vi "Autonomous Independent.vi"() -> ()   [LabVIEW 2015]
doc: "This VI is called when autonomous begins, and will automatically be terminated when autonomous ends. You can carry out timed or sensor driven robot movement independently without needing to return to the caller."
uses:
  <vilib>/Rock Robotics/WPI/Relay/WPI_RelayValue.ctl
  <vilib>/Rock Robotics/Network Tables/NT Read String.vi
  Robot Global Data.vi
  navX Library v2/navX Library v2.lvlib
panel:
  in  "Routine 2 - Shoot Encoder 2":dbl=1.78
  in  "Routine 2 - Shoot Encoder":dbl=1.78
  in  "Routine 1 - Target Angle":dbl=58.0
  in  "Routine 1 - Shoot Distance":dbl=16.0
  in  "Low Bar Height":dbl=1.2
  in  "Routine 1 - Shoot Encoder":dbl=1.63
  # "Actual distance for routine 1 is 17.5 ft"
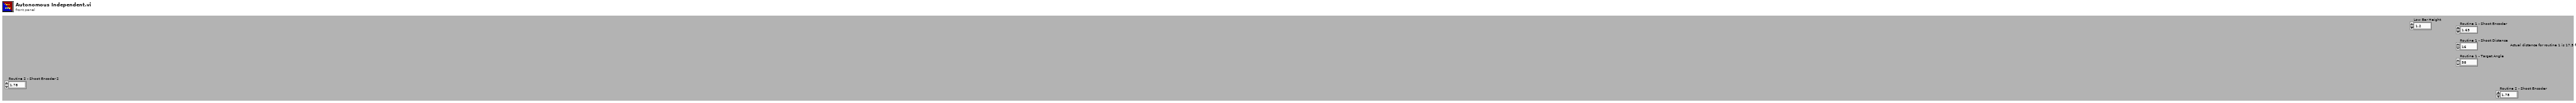
[diagram p1: front panel]
types:
  T1 = typedef "WPI_RelayValue.ctl" = enum16{"Off", "On", "Forward", "Reverse"}
  T2 = typedef "navX Library v2.lvlib/Z900_navX_DeviceTypeDef.ctl" = cluster{"Interface":cluster{"Protocol":T3, "Update Rate (4Hz-60Hz)":u8, "navX Open TypeDef":variant}, "Notify Packet":refnum<notifier>, "Loop VI Refnum":refnum<vi>, "Ready to Close Occurrence Refnum":refnum<k4>}
  T3 = typedef "navX Library v2.lvlib/Z900_navX_ProtocolTypeDef.ctl" = enum16{"SERIAL", "I2C", "SPI"}
  T4 = typedef "WPI_EncoderDevRef.ctl" = cluster{"DevStatus":errorcluster, "EncoderIndex":T5, "CounterIndex":T6, "DistancePerCount":dbl, "Decoding Type":T7}
  T5 = typedef "FPGA_EncoderIdx.ctl" = enum8{"Enc 0", "Enc 1", "Enc 2", "Enc 3", "Enc 4", "Enc 5", "Enc 6", "Enc 7", "Invalid"}
  T6 = typedef "FPGA_CounterCtrSystemIndex.ctl" = enum8{"Ctr 0", "Ctr 1", "Ctr 2", "Ctr 3", "Ctr 4", "Ctr 5", "Ctr 6", "Ctr 7", "Invalid"}
  T7 = typedef "WPI_EncoderType.ctl" = enum16{"1x", "2x", "4x"}
  T8 = typedef "WPI_RelayDevRef.ctl" = cluster{"DevStatus":errorcluster, "Relay Channel":T9, "Relay Direction":T10}
  T9 = typedef "FPGA_DIORelayChannel.ctl" = enum8{"Relay 0", "Relay 1", "Relay 2", "Relay 3", "Invalid"}
  T10 = typedef "WPI_RelayDirection.ctl" = enum16{"Both directions", "Forward only", "Reverse only"}
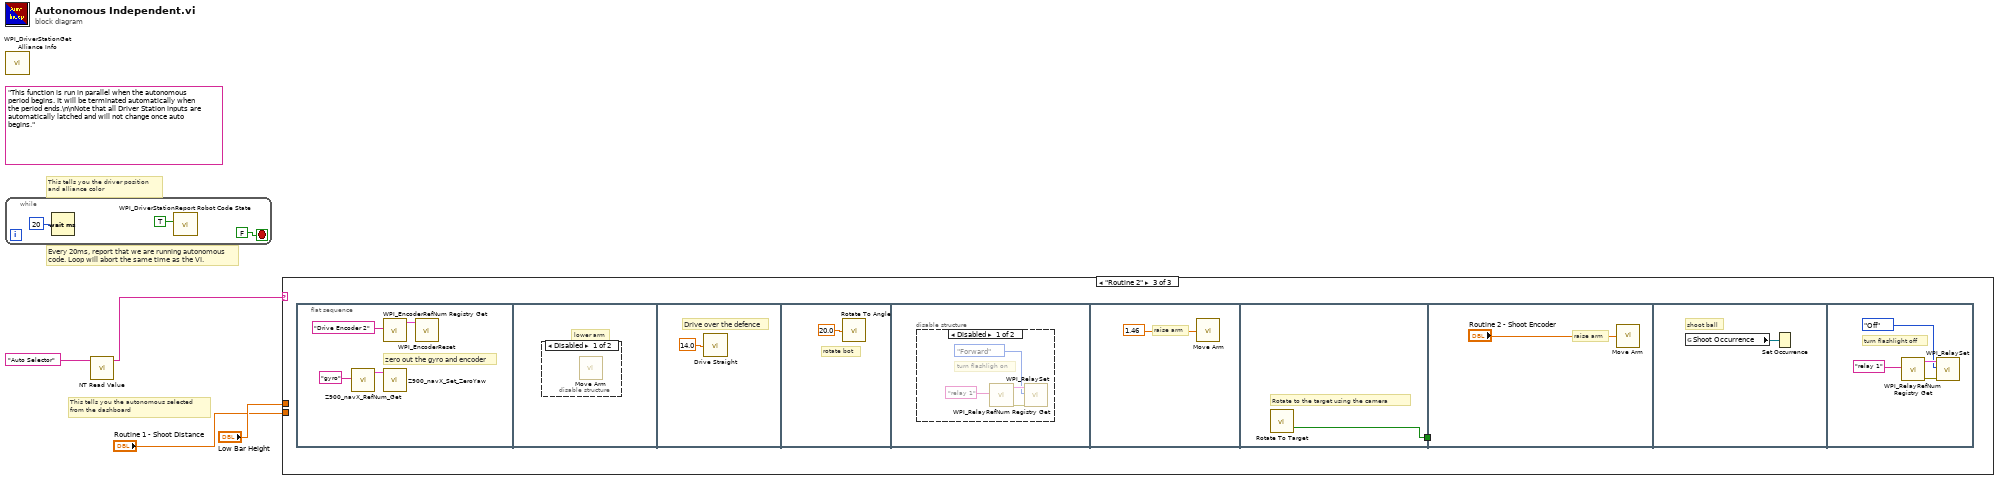
[diagram p0: block diagram]
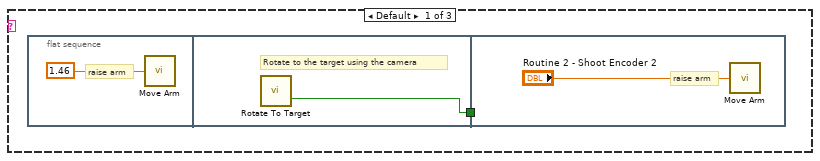
[diagram p2: hidden frame]
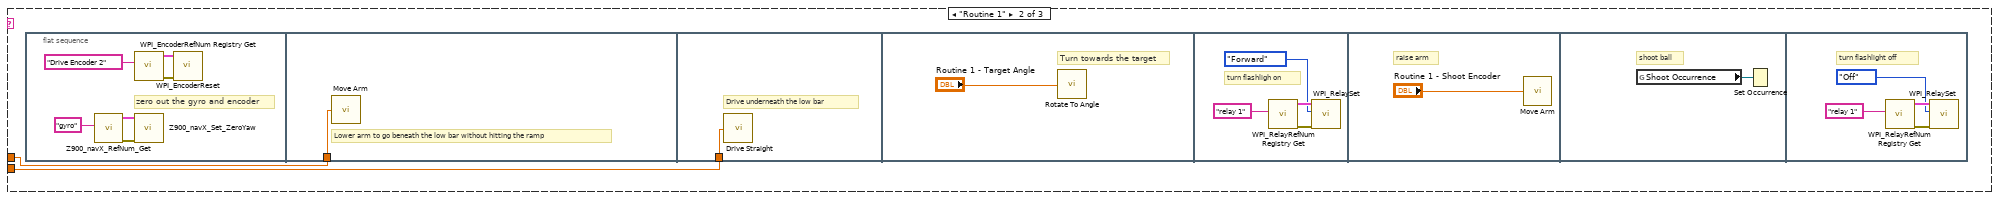
[diagram p3: hidden frame]
diagram:
  (unwired) "This function is run in parallel when the autonomous period begins. It will be terminated automatically when the period ends.\n\nNote that all Driver Station inputs are automatically latched and will not change once auto begins."
  # "This tells you the autonomous selected\nfrom the dashboard"
  # "Every 20ms, report that we are running autonomous\ncode. Loop will abort the same time as the VI."
  # "This tells you the driver position\nand alliance color"
  n1 = call <vilib>:"WPI_DriverStationGet Alliance Info.vi"() -> ()  [unwired: 12 out]
  n2 = while {
    stop <- FALSE stop-if-true
    n3 = Wait (ms)(milliseconds to wait=u32 20) -> ()  [unwired: 1 out]
    n4 = call <vilib>:"WPI_DriverStationReport Robot Code State.vi"("Autonomous"=TRUE) -> ()  [unwired: 10 in, 1 out]
  }
  n5 = call-poly <vilib>:"NT Read Value.vi"("Name"="Auto Selector") -> ("String"=w3:string)  [unwired: 9 in, 1 out]
  n6 = case shown="\"Routine 2\"" w3 {
    tunnel: "Low Bar Height" -> [_ w13 _]
    tunnel: "Routine 1 - Shoot Distance" -> [_ w12 _]
    frame Default {
      n7 = flat-sequence {
        tunnel: [w10] -> w8
        tunnel: w8 -> [_]
        frame #0 {
          # "raise arm"
          n8 = call "Move Arm.vi"("Target Voltage"=1.46 ("y")) -> ()
        }
        frame #1 {
          # "Rotate to the target using the camera"
          n9 = call "Rotate To Target.vi"() -> ("On Target"=w10:bool)
        }
        frame #2 {
          # "raise arm"
          n10 = call "Move Arm.vi"("Target Voltage"="Routine 2 - Shoot Encoder 2") -> ()
        }
      }
    }
    frame "Routine 1" {
      n11 = flat-sequence {
        tunnel: w13 -> [w20]
        tunnel: w12 -> [w21]
        frame #0 {
          # "zero out the gyro and encoder"
          n12 = call "Z900_navX_RefNum_Get.vi"("refnum name"="gyro") -> ("error out"=w16:errorcluster, "navX Device"=w19:T2)  [unwired: 9 in]
          n13 = call <vilib>:"WPI_EncoderRefNum Registry Get.vi"("refnum name"="Drive Encoder 2") -> ("error out"=w14:errorcluster, "EncoderDevRef"=w18:T4)  [unwired: 9 in]
          n14 = call "Z900_navX_Set_ZeroYaw.vi"("error in (no error)"=w16, "navX Device"=w19) -> ()  [unwired: 8 in, 2 out]
          n15 = call <vilib>:"WPI_EncoderReset.vi"("error in (no error)"=w14, "EncoderDevRef"=w18) -> ()  [unwired: 8 in, 2 out]
        }
        frame #1 {
          # "Lower arm to go beneath the low bar without hitting the ramp"
          n16 = call "Move Arm.vi"("Target Voltage"=w20) -> ()
        }
        frame #2 {
          # "Drive underneath the low bar"
          n17 = call "Drive Straight.vi"("Distance (ft)"=w21) -> ()
        }
        frame #3 {
          # "Turn towards the target"
          n18 = call "Rotate To Angle.vi"("Angle (degrees)"="Routine 1 - Target Angle") -> ()
        }
        frame #4 {
          # "turn flashligh on"
          n19 = call <vilib>:"WPI_RelayRefNum Registry Get.vi"("refnum name"="relay 1") -> ("error out"=w24:errorcluster, "RelayDevRef"=w25:T8)  [unwired: 9 in]
          n20 = call <vilib>:"WPI_RelaySet.vi"("error in (no error)"=w24, "RelayValue"=WPI_RelayValue."Forward", "RelayDevRef"=w25) -> ()  [unwired: 7 in, 2 out]
        }
        frame #5 {
          # "raise arm"
          n21 = call "Move Arm.vi"("Target Voltage"="Routine 1 - Shoot Encoder") -> ()
        }
        frame #6 {
          # "shoot ball"
          n22 = global read "Robot Global Data.vi" "Shoot Occurrence"() -> (w28:refnum<k4>)
          n23 = Set Occurrence(w28) -> ()
        }
        frame #7 {
          # "turn flashlight off"
          n24 = call <vilib>:"WPI_RelayRefNum Registry Get.vi"("refnum name"="relay 1") -> ("error out"=w30:errorcluster, "RelayDevRef"=w31:T8)  [unwired: 9 in]
          n25 = call <vilib>:"WPI_RelaySet.vi"("error in (no error)"=w30, "RelayValue"=WPI_RelayValue."Off", "RelayDevRef"=w31) -> ()  [unwired: 7 in, 2 out]
        }
      }
    }
    frame "Routine 2" {
      n26 = flat-sequence {
        tunnel: [w45] -> w33
        tunnel: w33 -> [_]
        frame #0 {
          # "zero out the gyro and encoder"
          n27 = call "Z900_navX_RefNum_Get.vi"("refnum name"="gyro") -> ("navX Device"=w37:T2)  [unwired: 9 in, 1 out]
          n28 = call <vilib>:"WPI_EncoderRefNum Registry Get.vi"("refnum name"="Drive Encoder 2") -> ("EncoderDevRef"=w36:T4)  [unwired: 9 in, 1 out]
          n29 = call "Z900_navX_Set_ZeroYaw.vi"("navX Device"=w37) -> ()  [unwired: 9 in, 2 out]
          n30 = call <vilib>:"WPI_EncoderReset.vi"("EncoderDevRef"=w36) -> ()  [unwired: 9 in, 2 out]
        }
        frame #1 {
          # "lower arm"
          n31 = disable-structure shown="Disabled" {
            frame Disabled {
              n32 = call "Move Arm.vi"() -> ()  [unwired: 1 in]
            }
            frame Enabled {
            }
          }
        }
        frame #2 {
          # "Drive over the defence"
          n33 = call "Drive Straight.vi"("Distance (ft)"=14.0 ("t")) -> ()
        }
        frame #3 {
          # "rotate bot"
          n34 = call "Rotate To Angle.vi"("Angle (degrees)"=20.0 ("t")) -> ()
        }
        frame #4 {
          n35 = disable-structure shown="Disabled" {
            frame Disabled {
              # "turn flashligh on"
              n36 = call <vilib>:"WPI_RelayRefNum Registry Get.vi"("refnum name"="relay 1") -> ("error out"=w41:errorcluster, "RelayDevRef"=w42:T8)  [unwired: 9 in]
              n37 = call <vilib>:"WPI_RelaySet.vi"("error in (no error)"=w41, "RelayValue"=WPI_RelayValue."Forward", "RelayDevRef"=w42) -> ()  [unwired: 7 in, 2 out]
            }
            frame Enabled {
            }
          }
        }
        frame #5 {
          # "raise arm"
          n38 = call "Move Arm.vi"("Target Voltage"=1.46 ("y")) -> ()
        }
        frame #6 {
          # "Rotate to the target using the camera"
          n39 = call "Rotate To Target.vi"() -> ("On Target"=w45:bool)
        }
        frame #7 {
          # "raise arm"
          n40 = call "Move Arm.vi"("Target Voltage"="Routine 2 - Shoot Encoder") -> ()
        }
        frame #8 {
          # "shoot ball"
          n41 = global read "Robot Global Data.vi" "Shoot Occurrence"() -> (w47:refnum<k4>)
          n42 = Set Occurrence(w47) -> ()
        }
        frame #9 {
          # "turn flashlight off"
          n43 = call <vilib>:"WPI_RelayRefNum Registry Get.vi"("refnum name"="relay 1") -> ("error out"=w49:errorcluster, "RelayDevRef"=w50:T8)  [unwired: 9 in]
          n44 = call <vilib>:"WPI_RelaySet.vi"("error in (no error)"=w49, "RelayValue"=WPI_RelayValue."Off", "RelayDevRef"=w50) -> ()  [unwired: 7 in, 2 out]
        }
      }
    }
  }
